vi "PID_Gain_Converter.vi"() -> (3 "Cluster":cluster{dbl, dbl, dbl}={1.0, 0.001, 0.0})   [LabVIEW 2017]
panel:
  in  "Derivative":dbl
  in  "Integral":dbl=0.67
  in  "Proportional":dbl=14.0
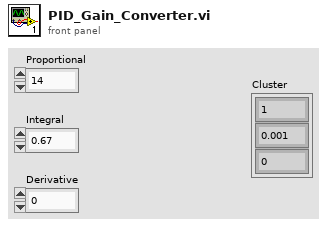
[diagram p1: front panel]
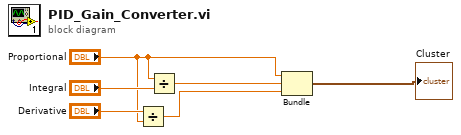
[diagram p0: block diagram]
diagram:
  n1 = Divide(x="Derivative", y="Proportional") -> (x/y=w1:dbl)
  n2 = Divide(x="Proportional", y="Integral") -> (x/y=w4:dbl)
  n3 = Bundle("Proportional"="Proportional", w4, w1) -> (→"Cluster":cluster{"Proportional":dbl, dbl, dbl})  [unwired: 1 in]
